vi "CMC_Clean.vi"() -> ()   [LabVIEW 2013]
doc: "A sample VI demonstrating a pooly designed front panel and block diagram."
panel:
  in  "Math Functions":enum32{"Add", "Multiply"}(tab)
  in  "X":dbl
  in  "Y":dbl
  out "Result":dbl
  in  "X":dbl
  in  "Y":dbl
  out "Result":dbl
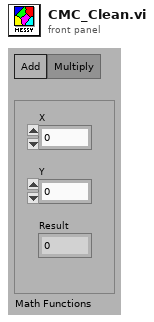
[diagram p1: front panel]
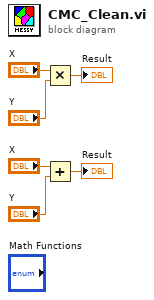
[diagram p0: block diagram]
diagram:
  n1 = Multiply(x="X", y="Y") -> (x*y=→"Result":dbl)
  n2 = Add(x="X", y="Y") -> (x+y=→"Result":dbl)
